vi "Register gRPC Methods.vi"(8 "error in (no error)":errorcluster, 11 "Template Server in":refnum<class "OCV3.lvclass">) -> (0 "error out":errorcluster, 3 "Template Server out":refnum<class "OCV3.lvclass">)   [LabVIEW 2019, in "OCV3.lvlib" / "OCV3.lvclass"]
uses:
  OCV3.lvclass
  typeDefs/Server Internal UEs.ctl
  typeDefs/Server Internal Message.ctl
  typeDefs/Server gRPC UEs.ctl
  gRPC lvSupport/Server API/typeDefs/gRPCId Cluster.ctl
  gRPC lvSupport/Server API/typeDefs/grpcId.ctl
  OCV3.lvclass/OCV3.ctl
  gRPC lvSupport/gprc-lvsupport.lvlib
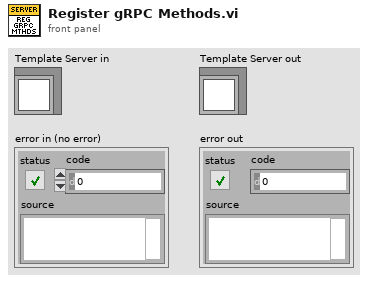
[diagram p1: front panel]
types:
  T1 = typedef "OCV3.lvlib/OCV3.lvclass/Server gRPC UEs.ctl" = cluster{"Invoke gRPC UE":refnum<user-event>, "Query gRPC UE":refnum<user-event>, "PerformOCVMeasurement gRPC UE":refnum<user-event>, "PerformACIRMeasurement gRPC UE":refnum<user-event>, "StreamOCVMeasurement gRPC UE":refnum<user-event>, "Register gRPC UE":refnum<user-event>}
  T2 = typedef "OCV3.lvlib/OCV3.lvclass/Server Internal UEs.ctl" = cluster{"Invoke Internal UE":refnum<user-event>, "Query Internal UE":refnum<user-event>, "PerformOCVMeasurement Internal UE":refnum<user-event>, "PerformACIRMeasurement Internal UE":refnum<user-event>, "StreamOCVMeasurement Internal UE":refnum<user-event>, "Register Internal UE":refnum<user-event>}
  T3 = typedef "OCV3.lvlib/gprc-lvsupport.lvlib/grpcId.ctl" = u64
  T4 = typedef "OCV3.lvlib/OCV3.lvclass/Server Internal Message UE.ctl" = refnum<user-event>
  T5 = typedef "OCV3.lvlib/gprc-lvsupport.lvlib/gRPCId Cluster UE.ctl" = refnum<user-event>
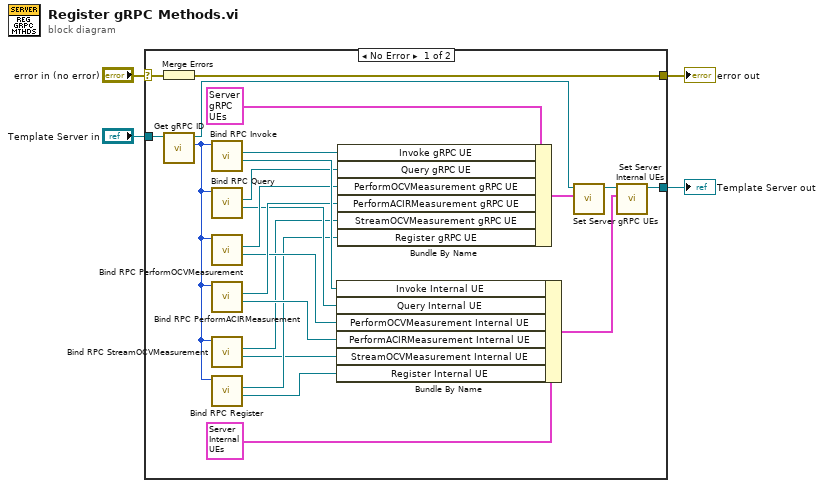
[diagram p0: block diagram]
diagram:
  n1 = case shown="No Error" "error in (no error)" {
    selector: "error in (no error)" -> [w18 w28]
    tunnel: "Template Server in" -> [w26 w29]
    tunnel: [w25 w28] -> w3
    tunnel: [w24 w29] -> w2
    frame No Error {
      n2 = Merge Errors(w18) -> (w25:errorcluster)
      n3 = call "Get gRPC ID.vi"("OOP Server in"=w26) -> ("gRPC ID"=w17:T3, "OOP Server out"=w27:refnum<class "OCV3.lvclass">)  [unwired: 9 in]
      n4 = call "Bind RPC Invoke.vi"("gRPCid server in"=w17) -> ("Invoke Internal UE"=w16:T4, "Invoke gRPC UE"=w15:T5)  [unwired: 7 in, 2 out]
      n5 = call "Bind RPC Query.vi"("gRPCid server in"=w17) -> ("Query Internal UE"=w10:T4, "Query gRPC UE"=w9:T5)  [unwired: 7 in, 2 out]
      n6 = call "Bind RPC PerformOCVMeasurement.vi"("gRPCid server in"=w17) -> ("PerformOCVMeasurement Internal UE"=w12:T4, "PerformOCVMeasurement gRPC UE"=w11:T5)  [unwired: 7 in, 2 out]
      n7 = call "Bind RPC PerformACIRMeasurement.vi"("gRPCid server in"=w17) -> ("PerformACIRMeasurement Internal UE"=w14:T4, "PerformACIRMeasurement gRPC UE"=w13:T5)  [unwired: 7 in, 2 out]
      n8 = call "Bind RPC StreamOCVMeasurement.vi"("gRPCid server in"=w17) -> ("StreamOCVMeasurement Internal UE"=w6:T4, "StreamOCVMeasurement gRPC UE"=w5:T5)  [unwired: 7 in, 2 out]
      n9 = call "Bind RPC Register.vi"("gRPCid server in"=w17) -> ("Register Internal UE"=w8:T4, "Register gRPC UE"=w7:T5)  [unwired: 7 in, 2 out]
      n10 = Bundle By Name ("Bundle Internal UEs")(cluster=T2 {"Invoke Internal UE"=refnum, "Query Internal UE"=refnum, "PerformOCVMeasurement Internal UE"=refnum, "PerformACIRMeasurement Internal UE"=refnum, "StreamOCVMeasurement Internal UE"=refnum, "Register Internal UE"=refnum} ("Server Internal UEs"), "Invoke Internal UE"=w16, "Query Internal UE"=w10, "PerformOCVMeasurement Internal UE"=w12, "PerformACIRMeasurement Internal UE"=w14, "StreamOCVMeasurement Internal UE"=w6, "Register Internal UE"=w8) -> (w23:T2)
      n11 = Bundle By Name ("Bundle gRPC UEs")(cluster=T1 {"Invoke gRPC UE"=refnum, "Query gRPC UE"=refnum, "PerformOCVMeasurement gRPC UE"=refnum, "PerformACIRMeasurement gRPC UE"=refnum, "StreamOCVMeasurement gRPC UE"=refnum, "Register gRPC UE"=refnum} ("gRPC Server Method Events"), "Invoke gRPC UE"=w15, "Query gRPC UE"=w9, "PerformOCVMeasurement gRPC UE"=w11, "PerformACIRMeasurement gRPC UE"=w13, "StreamOCVMeasurement gRPC UE"=w5, "Register gRPC UE"=w7) -> (w20:T1)
      n12 = call "Set Server gRPC UEs.vi"("Server gRPC UEs"=w20, "OOP Server in"=w27) -> ("OOP Server out"=w21:refnum<class "OCV3.lvclass">)  [unwired: 9 in]
      n13 = call "Set Server Internal UEs.vi"("Server Internal UEs"=w23, "OOP Server in"=w21) -> ("OOP Server out"=w24:refnum<class "OCV3.lvclass">)  [unwired: 9 in]
    }
    frame Error {
    }
  }
  "error out" <- w3
  "Template Server out" <- w2
